vi "constant vi validation.vi"(9 "Constant VI Arg window":refnum<vi>, 10 "New Constant vi name":string, 11 "Constant VI":string[](array[string])) -> (3 "No Error Duplication":bool)   [LabVIEW 2019, in "Panther Dashboard.lvlib"]
uses:
  Panther Dashboard.lvlib
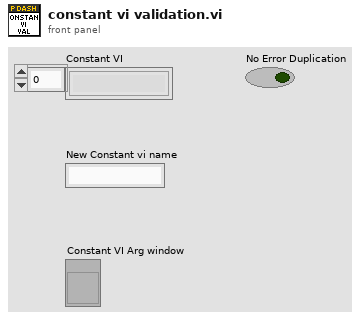
[diagram p1: front panel]
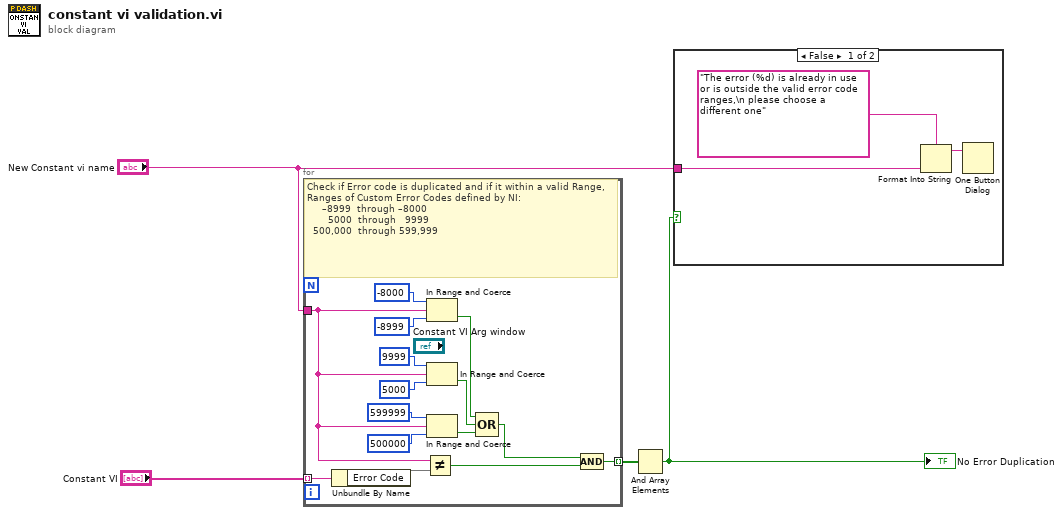
[diagram p0: block diagram]
diagram:
  n1 = for {
    tunnel: "Constant VI" -> [w19] mode=indexing
    tunnel: "New Constant vi name" -> [w11]
    tunnel: [w10] -> w4 mode=indexing
    # "Check if Error code is duplicated and if it within a valid Range,\nRanges of Custom Error Codes defined by NI:\n     –8999  through –8000\n       5000  through   9999\n  500,000  through 599,999"
    n2 = Unbundle By Name(w19) -> ("Error Code"=w18)
    n3 = Not Equal?(x=w11, y=w18) -> (x != y?=w6:bool)
    n4 = In Range and Coerce(upper limit=-8000, x=w11, lower limit=-8999 ("upper limit")) -> (In Range?=w9:bool)  [unwired: 1 out]
    n5 = In Range and Coerce(upper limit=9999, x=w11, lower limit=5000 ("upper limit")) -> (In Range?=w8:bool)  [unwired: 1 out]
    n6 = In Range and Coerce(upper limit=599999, x=w11, lower limit=500000 ("upper limit")) -> (In Range?=w7:bool)  [unwired: 1 out]
    n7 = Compound Arithmetic op=OR(w9, w8, w7) -> (w5:bool)
    n8 = Compound Arithmetic op=AND(w5, w6) -> (w10:bool)
  }
  n9 = And Array Elements(Boolean array=w4) -> (logical AND=w1:bool)
  "No Error Duplication" <- w1
  n10 = case shown="False" w1 {
    tunnel: "New Constant vi name" -> [w21 _]
    frame False {
      n11 = Format Into String(format string="The error (%d) is already in use or is outside the valid error code ranges,\n please choose a different one", w21) -> (resulting string=w22:string)  [unwired: 2 in, 1 out]
      n12 = One Button Dialog(message=w22) -> ()  [unwired: 1 in, 1 out]
    }
    frame True {
    }
  }
